vi "RESTful INI Update Body Tag.vi"(6 "Tag":string, 8 "error in (no error)":errorcluster, 10 "Replacement String":string, 11 "Input String":string) -> (0 "error out":errorcluster, 3 "result string":string)   [LabVIEW 2020]
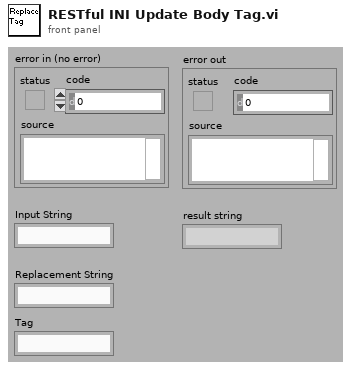
[diagram p1: front panel]
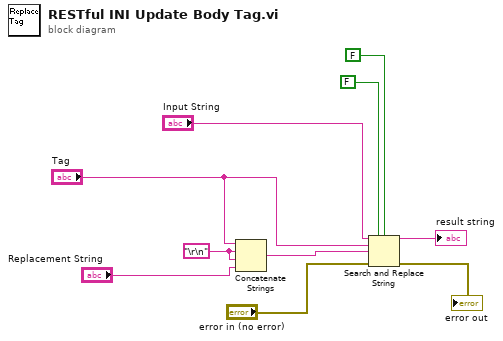
[diagram p0: block diagram]
diagram:
  w5 = "\r\n"
  n1 = Concatenate Strings("Tag", w5, w5, "Replacement String") -> (w7:string)
  n2 = Search and Replace String(replace all?=FALSE ("replace all? (F)"), case sensitive?=FALSE ("ignore case? (F)"), input string="Input String", search string="Tag", replace string=w7, error in="error in (no error)") -> (result string=→"result string":string, error out=→"error out":errorcluster)  [unwired: 4 out]
